vi "ChannelSet.vi"(6 "设置参数":string, 7 "参数查询(0)/设置(1)":bool, 8 "error in (no error)":errorcluster caption="错误输入（无错误）", 9 "CHANNLE命令子系统":string(combo), 10 "通道选择":string(combo), 11 "VISA资源名称":refnum<visa-resource-name>) -> (0 "error out":errorcluster caption="错误输出", 1 "查询返回字节数":u32, 2 "查询返回":string, 3 "VISA资源名称 2":refnum<visa-resource-name>)   [LabVIEW 2018]
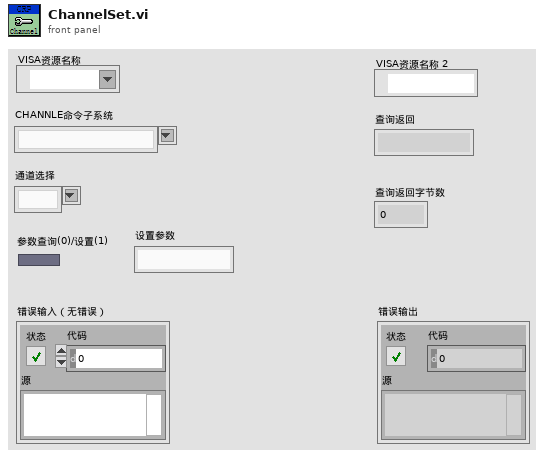
[diagram p1: front panel]
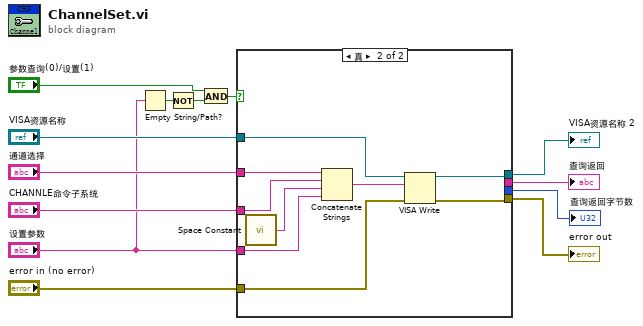
[diagram p0: block diagram]
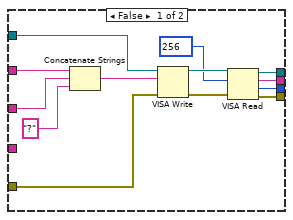
[diagram p2: hidden frame]
diagram:
  n1 = Empty String/Path?(string/path="设置参数") -> (empty?=w6:bool)
  n2 = Not(x=w6) -> (.not. x?=w1:bool)
  n3 = And(x="参数查询(0)/设置(1)", y=w1) -> (x .and. y?=w4:bool)
  n4 = case shown="真" w4 {
    tunnel: "设置参数" -> [_ w35]
    tunnel: "通道选择" -> [w26 w33]
    tunnel: "CHANNLE命令子系统" -> [w25 w32]
    tunnel: "VISA资源名称" -> [w22 w31]
    tunnel: "error in (no error)" -> [w21 w29]
    tunnel: [w17 w27] -> w7
    tunnel: [w16 w28] -> w8
    tunnel: [w15 _] -> w9
    tunnel: [w14 _] -> w2
    frame False {
      n5 = Concatenate Strings(w26, w25, "?" ("字符串")) -> (w23:string)
      n6 = VISA Write(VISA resource name=w22, write buffer=w23, error in (no error)=w21) -> (VISA resource name out=w20:refnum<visa-resource-name>, error out=w19:errorcluster)  [unwired: 1 out]
      n7 = VISA Read(VISA resource name=w20, byte count=u32 256 ("字节总数"), error in (no error)=w19) -> (VISA resource name out=w16:refnum<visa-resource-name>, read buffer=w15:string, return count=w14:u32, error out=w17:errorcluster)
    }
    frame True {
      n8 = call <vilib>:"Space Constant.vi"() -> ("String"=w34:string)
      n9 = Concatenate Strings(w33, w32, w34, w35) -> (w30:string)
      n10 = VISA Write(VISA resource name=w31, write buffer=w30, error in (no error)=w29) -> (VISA resource name out=w28:refnum<visa-resource-name>, error out=w27:errorcluster)  [unwired: 1 out]
    }
  }
  "VISA资源名称 2" <- w8
  "error out" <- w7
  "查询返回" <- w9
  "查询返回字节数" <- w2
